vi "FORMat.vi"(8 "error in (no error)":errorcluster, 10 "Function":T1(ring), 11 "VISA resource":refnum<visa-resource-name>) -> (0 "error out":errorcluster, 2 "Response":string, 3 "Dup VISA resource":refnum<visa-resource-name>)   [LabVIEW 2010]
doc: "Copyright (c) 2012 Metrolab Technology SA, Plan-les-Ouates, Geneva, Switzerland\nSets the output format for measurements, or gets the current setting. The output format can be text (ÒASCiiÓ), uncompressed binary (ÒINTegerÓ), or compressed binary (\"PACKed1\" or \"PACKed2\"). The output format is further affected by the CALibration:STATe and UNIT settings:\n- FORM=ASC, CAL:STAT=ON:\n Measurement in text, selected units\n- FORM=ASC, CAL:STAT=OFF:\n Measurement in text, raw ADC values\n- FORM=INT, CAL:STAT=ON:\n Measurement in 32-bit binary, µT\n- FORM=INT, CAL:STAT=OFF:\n Measurement in 32-bit binary, raw ADC values\n- FORM=PACKed1, CAL:STAT=ON:\n Measurement in 8-bit binary delta, µT\n- FORM=PACKed1, CAL:STAT=OFF:\n Measurement in 8-bit binary delta, raw ADC values\n- FORM=PACKed2, CAL:STAT=ON:\n Measurement in 16-bit binary delta, µT\n- FORM=PACKed2, CAL:STAT=OFF:\n Measurement in 16-bit binary delta, raw ADC values\nNote that MEASure_FETCh_READ parses binary, packed as well as text output."
panel:
  # "FORMat"
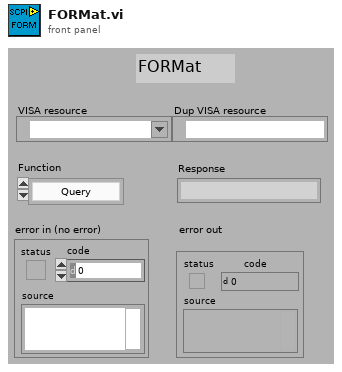
[diagram p1: front panel]
types:
  T1 = enum16{"Query", "ASCii", "INTeger", "PACKed1", "PACKed2"}
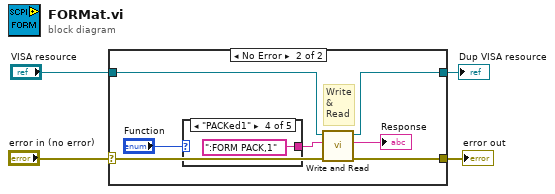
[diagram p0: block diagram]
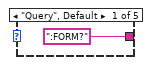
[diagram p3: hidden frame]
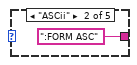
[diagram p4: hidden frame]
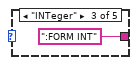
[diagram p5: hidden frame]
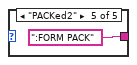
[diagram p6: hidden frame]
diagram:
  n1 = case shown="No Error" "error in (no error)" {
    selector: "error in (no error)" -> [w6 w12]
    tunnel: [w6 w11] -> w4
    tunnel: [w5 w8] -> w2
    tunnel: "VISA resource" -> [w5 w7]
    frame Error {
    }
    frame No Error {
      # "Write\n&\nRead"
      n2 = case shown="\"PACKed1\"" "Function" {
        tunnel: [":FORM?" ":FORM ASC" ":FORM INT" ":FORM PACK,1" ":FORM PACK"] -> w9
        frame "Query", Default {
        }
        frame "ASCii" {
        }
        frame "INTeger" {
        }
        frame "PACKed1" {
        }
        frame "PACKed2" {
        }
      }
      n3 = call "Write and Read.vi"("Error in (no error)"=w12, "Command"=w9, "VISA resource"=w7) -> ("Error out"=w11:errorcluster, "Response"=→"Response":string, "Dup VISA resource"=w8:refnum<visa-resource-name>)  [unwired: 4 in, 2 out]
    }
  }
  "error out" <- w4
  "Dup VISA resource" <- w2
